vi "Get Exposure Range.vi"(8 "error in (no error)":errorcluster) -> (0 "error out":errorcluster, 1 "Exp Range Max":u32, 2 "Exp Range Min":u32)   [LabVIEW 2017]
doc: "Returns the maximum and minimum available exposure values in ms."
uses:
  WLM variable typedefs.llb/Exposure range.ctl
  HighFinesse WS5/wlmData.dll
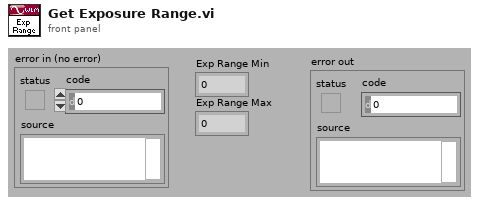
[diagram p1: front panel]
types:
  T1 = typedef "Exposure range.ctl" = i16
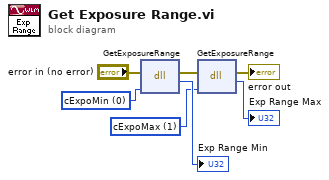
[diagram p0: block diagram]
diagram:
  w4 = T1 1 items=["cExpoMin", "cExpoMax", "cExpo2Min", "cExpo2Max"] ("Exposure range constants")
  w6 = T1 0 items=["cExpoMin", "cExpoMax", "cExpo2Min", "cExpo2Max"] ("Exposure range constants")
  n1 = dll-call lib="C:/LabVIEW-programs-dev/Instruments/Wavelength meter/HighFinesse WS5/wlmData.dll" fn="GetExposureRange"(error in="error in (no error)", "ER"=w6) -> (error out=w2:errorcluster, "return type"=→"Exp Range Min":u32)  [unwired: 3 in, 1 out]
  n2 = dll-call lib="C:/LabVIEW-programs-dev/Instruments/Wavelength meter/HighFinesse WS5/wlmData.dll" fn="GetExposureRange"(error in=w2, "ER"=w4) -> (error out=→"error out":errorcluster, "return type"=→"Exp Range Max":u32)  [unwired: 3 in, 1 out]
